vi "Condition Name Msg IO.vi"(4 "IO":T2, 6 "Terminals (All)":T1, 8 "error in":errorcluster, 9 "Name Msg IO":T5, 10 "Name jettl Msg.Name VI (Interface)":refnum<vi>) -> (0 "error out":errorcluster, 1 "Terminal Attributes (Read)":T3, 2 "Terminal Attributes (Init)":T3)   [LabVIEW 2020, in "_Rescript.lvlib" / "Msg.lvlib" / "Msg.lvclass"]
uses:
  Msg.lvclass
  Name Msg IO.ctl
  Terminal Attributes.ctl
  Attributes.ctl
  IO.ctl
  Terminals.ctl
  <vilib>/Utility/traverseref.llb/TRef TravTarget.ctl
  _Rescript.lvlib
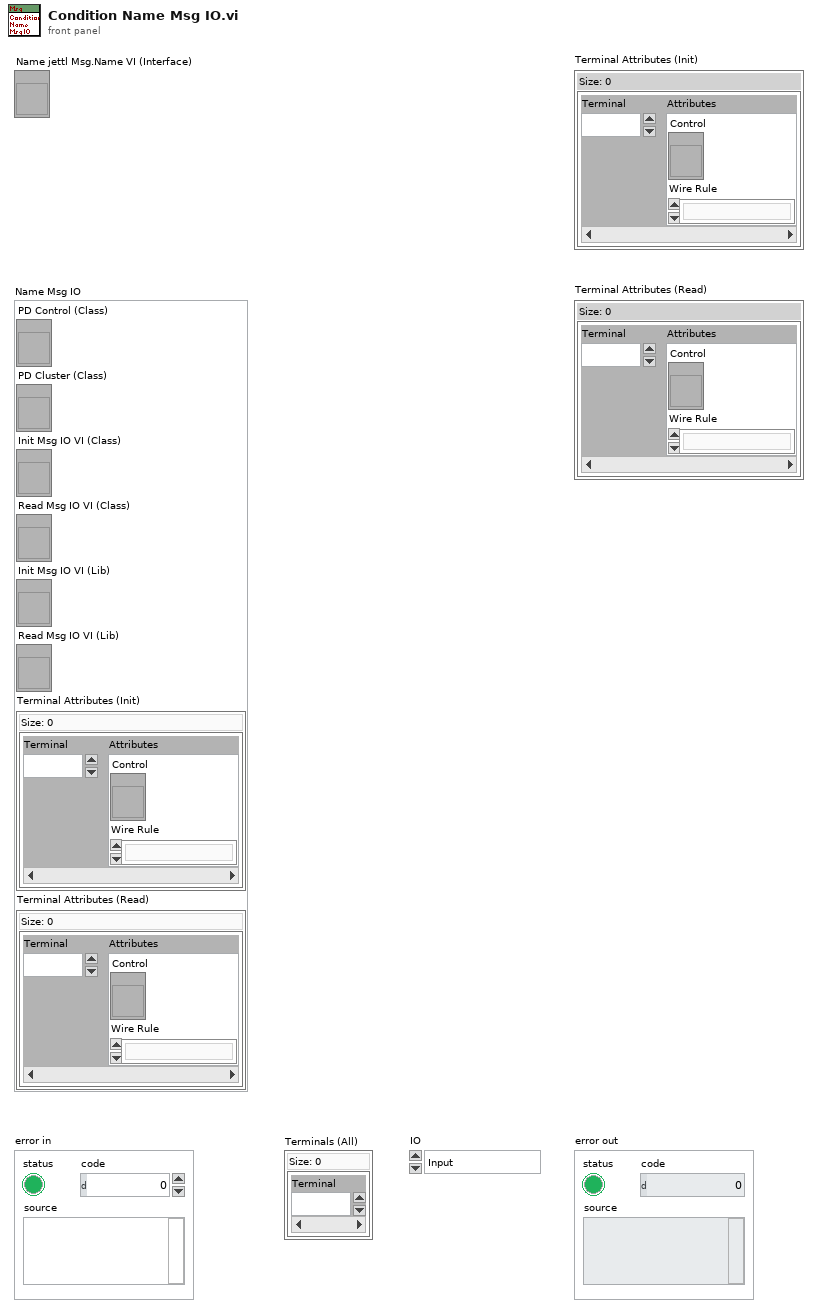
[diagram p1: front panel]
types:
  T1 = typedef "_Rescript.lvlib/Terminals.ctl" = set{i32}
  T2 = typedef "_Rescript.lvlib/Msg.lvlib/Msg.lvclass/IO.ctl" = enum16{"Input", "Output"}
  T3 = typedef "_Rescript.lvlib/Terminal Attributes.ctl" = map{i32, T4}
  T4 = typedef "_Rescript.lvlib/Attributes.ctl" = cluster{"Control":refnum<vi>, "Wire Rule":enum16{"Invalid Wire Rule", "Required", "Recommended", "Optional", "Dynamic Dispatch"}}
  T5 = typedef "_Rescript.lvlib/Msg.lvlib/Msg.lvclass/Name Msg IO.ctl" = cluster{"PD Control (Class)":refnum<vi>, "PD Cluster (Class)":refnum<vi>, "Init Msg IO VI (Class)":refnum<vi>, "Read Msg IO VI (Class)":refnum<vi>, "Init Msg IO VI (Lib)":refnum<vi>, "Read Msg IO VI (Lib)":refnum<vi>, "Terminal Attributes (Init)":T3, "Terminal Attributes (Read)":T3}
  T6 = typedef "TRef TravTarget.ctl" = enum16{"FP", "BD", "Other"}
  T7 = typedef "_Rescript.lvlib/Msg.lvlib/Msg.lvclass/Terminal Relation.ctl" = map{i32, i32}
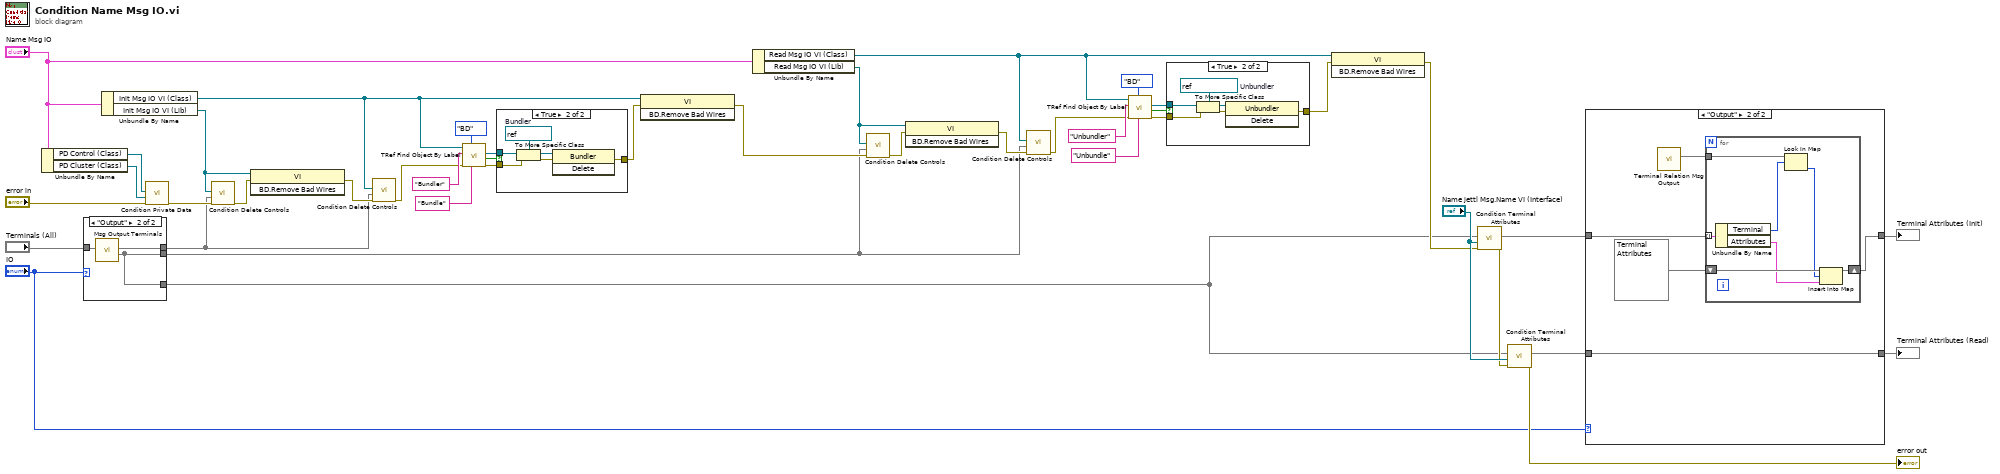
[diagram p0: block diagram]
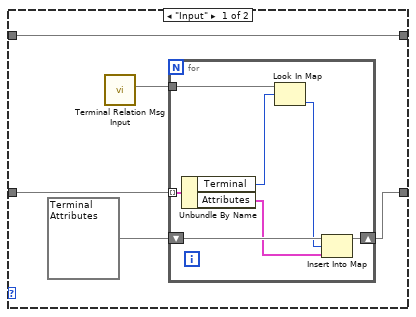
[diagram p2: hidden frame]
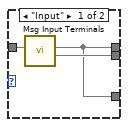
[diagram p3: hidden frame]
diagram:
  n1 = Unbundle By Name("Name Msg IO") -> ("PD Control (Class)"=w37:refnum<vi>, "PD Cluster (Class)"=w36:refnum<vi>)
  n2 = case shown="\"Output\"" "IO" {
    tunnel: "Terminals (All)" -> [w46 w49]
    tunnel: [w45 w47] -> w8
    tunnel: [w44 w48] -> w7
    tunnel: [w44 w47] -> w6
    frame "Input" {
      n3 = call "Msg Input Terminals.vi"("Terminals"=w46) -> ("Terminals (Read Msg Input)"=w45:T1, "Terminals (Init Msg Input)"=w44:T1)  [unwired: 9 in]
    }
    frame "Output" {
      n4 = call "Msg Output Terminals.vi"("Terminals (Msg Output)"=w49) -> ("Terminals (Read Msg Output)"=w47:T1, "Terminals (Init Msg Output)"=w48:T1)  [unwired: 9 in]
    }
  }
  n5 = Unbundle By Name("Name Msg IO") -> ("Init Msg IO VI (Class)"=w27:refnum<vi>, "Init Msg IO VI (Lib)"=w30:refnum<vi>)
  n6 = call "Condition Private Data.vi"("error in"="error in", "PD Cluster"=w36, "PD Control"=w37) -> ("error out"=w33:errorcluster)  [unwired: 8 in]
  n7 = call "Condition Delete Controls.vi"("error in"=w33, "Terminals"=w7, "VI"=w30) -> ("error out"=w32:errorcluster)  [unwired: 8 in]
  n8 = invoke class="VI" method="BD.Remove Bad Wires"(reference=w30, error in=w32) -> (error out=w31:errorcluster)  [unwired: 1 in, 2 out]
  n9 = call "Condition Delete Controls.vi"("error in"=w31, "Terminals"=w7, "VI"=w27) -> ("error out"=w38:errorcluster)  [unwired: 8 in]
  n10 = call <vilib>:"TRef Find Object By Label.vi"("Label"="Bundle", "Traverse Target"=TRef_TravTarget."BD", "error in (no error)"=w38, "Class Name"="Bundler", "VI Ref"=w27) -> ("error out"=w43:errorcluster, "Found?"=w11:bool, "Found Obj Ref"=w42:refnum<vi>)  [unwired: 3 in, 1 out]
  n11 = case shown="True" w11 {
    tunnel: w43 -> [w50 w56]
    tunnel: w42 -> [_ w54]
    tunnel: [w50 w52] -> w26
    frame False {
    }
    frame True {
      w55 = refnum<vi> refnum  # Bundler
      n12 = To More Specific Class(target class=w55, reference=w54, error in=w56) -> (specific class reference=w53:refnum<vi>, error out=w51:errorcluster)
      n13 = invoke class="Bundler" method="Delete"(reference=w53, error in=w51) -> (error out=w52:errorcluster)  [unwired: 1 in, 2 out]
    }
  }
  n14 = invoke class="VI" method="BD.Remove Bad Wires"(reference=w27, error in=w26) -> (error out=w13:errorcluster)  [unwired: 1 in, 2 out]
  n15 = Unbundle By Name("Name Msg IO") -> ("Read Msg IO VI (Class)"=w15:refnum<vi>, "Read Msg IO VI (Lib)"=w14:refnum<vi>)
  n16 = call "Condition Delete Controls.vi"("error in"=w13, "Terminals"=w8, "VI"=w14) -> ("error out"=w18:errorcluster)  [unwired: 8 in]
  n17 = invoke class="VI" method="BD.Remove Bad Wires"(reference=w14, error in=w18) -> (error out=w17:errorcluster)  [unwired: 1 in, 2 out]
  n18 = call "Condition Delete Controls.vi"("error in"=w17, "Terminals"=w8, "VI"=w15) -> ("error out"=w19:errorcluster)  [unwired: 8 in]
  n19 = call <vilib>:"TRef Find Object By Label.vi"("Label"="Unbundle", "Traverse Target"=TRef_TravTarget."BD", "error in (no error)"=w19, "Class Name"="Unbundler", "VI Ref"=w15) -> ("error out"=w24:errorcluster, "Found?"=w10:bool, "Found Obj Ref"=w23:refnum<vi>)  [unwired: 3 in, 1 out]
  n20 = case shown="True" w10 {
    tunnel: w24 -> [w57 w63]
    tunnel: w23 -> [_ w61]
    tunnel: [w57 w59] -> w16
    frame False {
    }
    frame True {
      w62 = refnum<vi> refnum  # Unbundler
      n21 = To More Specific Class(target class=w62, reference=w61, error in=w63) -> (specific class reference=w60:refnum<vi>, error out=w58:errorcluster)
      n22 = invoke class="Unbundler" method="Delete"(reference=w60, error in=w58) -> (error out=w59:errorcluster)  [unwired: 1 in, 2 out]
    }
  }
  n23 = invoke class="VI" method="BD.Remove Bad Wires"(reference=w15, error in=w16) -> (error out=w12:errorcluster)  [unwired: 1 in, 2 out]
  n24 = call "Condition Terminal Attributes.vi"("error in"=w12, "VI"="Name jettl Msg.Name VI (Interface)", "Terminals"=w6) -> ("error out"=w29:errorcluster, "Terminal Attributes"=w4:T3)  [unwired: 7 in]
  n25 = call "Condition Terminal Attributes.vi"("error in"=w29, "VI"="Name jettl Msg.Name VI (Interface)", "Terminals"=w6) -> ("error out"=→"error out":errorcluster, "Terminal Attributes"=w2:T3)  [unwired: 7 in]
  n26 = case shown="\"Output\"" "IO" {
    tunnel: [w68 w78] -> w5
    tunnel: w4 -> [w68 w77]
    tunnel: [w67 w80] -> w3
    tunnel: w2 -> [w66 w80]
    frame "Input" {
      n27 = call "Terminal Relation Msg Input.vi"() -> ("Terminal Relation (Msg Input)"=w64:T7)  [unwired: 11 in]
      n28 = for {
        shift-right: [w73] -> w67
        shift-left: T3 {} ("Terminal Attributes") -> [w74]
        tunnel: w66 -> [w75] mode=indexing
        tunnel: w64 -> [w71]
        n29 = Unbundle By Name(w75) -> ("Terminal"=w69:i32, "Attributes"=w72:T4)
        n30 = Look In Map(map=w71, key=w69) -> (value=w70:i32)  [unwired: 1 in, 1 out]
        n31 = Insert Into Map(map in=w74, key=w70, value=w72) -> (map out=w73:T3)  [unwired: 2 out]
      }
    }
    frame "Output" {
      n32 = call "Terminal Relation Msg Output.vi"() -> ("Terminal Relation (Msg Output)"=w76:T7)  [unwired: 11 in]
      n33 = for {
        shift-right: [w85] -> w78
        shift-left: T3 {} ("Terminal Attributes") -> [w86]
        tunnel: w77 -> [w87] mode=indexing
        tunnel: w76 -> [w83]
        n34 = Unbundle By Name(w87) -> ("Terminal"=w81:i32, "Attributes"=w84:T4)
        n35 = Look In Map(map=w83, key=w81) -> (value=w82:i32)  [unwired: 1 in, 1 out]
        n36 = Insert Into Map(map in=w86, key=w82, value=w84) -> (map out=w85:T3)  [unwired: 2 out]
      }
    }
  }
  "Terminal Attributes (Init)" <- w5
  "Terminal Attributes (Read)" <- w3
